vi "LoadPluginRequest.vi"(8 "error in (no error)":errorcluster, 10 "PathToPlugin":path=path "", 11 "ModuleID":i32=-1) -> (0 "error out":errorcluster)   [LabVIEW 2014, in "EventModule.lvlib"]
uses:
  EventModule.lvlib
  clEventType.ctl
  <vilib>/Utility/error.llb/Error Cluster From Error Code.vi
  <vilib>/ErrorRing/Error Ring.xnode
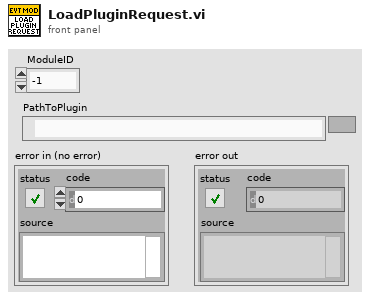
[diagram p1: front panel]
types:
  T1 = typedef "EventModule.lvlib/clRequestEvents.ctl" = cluster{"StopRequest":refnum<user-event>, "LoadPluginRequest":refnum<user-event>, "WriteEvtConfig":refnum<user-event>, "ReadEvtConfig":refnum<user-event>, "WriteTimeArray":refnum<user-event>, "ReadTimeArray":refnum<user-event>, "WriteEvtParams":refnum<user-event>, "ReadEvtParams":refnum<user-event>, "GetEvtReportArray":refnum<user-event>, "ReadPathToPlugin":refnum<user-event>, "GetEvtSignal":refnum<user-event>, "WriteBusNumber":refnum<user-event>, "ReadBusNumber":refnum<user-event>, "ShowPanel":refnum<user-event>}
  T2 = typedef "EventModule.lvlib/clEventType.ctl" = cluster{"ModuleID":i32, "Data":variant}
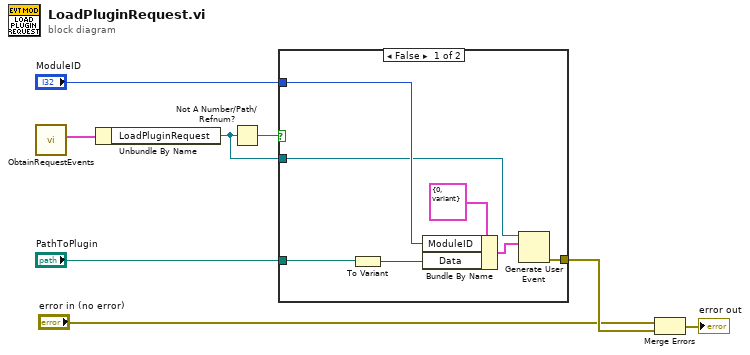
[diagram p0: block diagram]
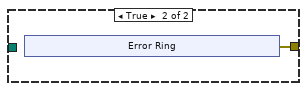
[diagram p2: hidden frame]
diagram:
  n1 = call "ObtainRequestEvents.vi"() -> ("clRequestEvents"=w8:T1)  [unwired: 10 in, 1 out]
  n2 = Unbundle By Name(w8) -> ("LoadPluginRequest"=w6:refnum<user-event>)
  n3 = Not A Number/Path/Refnum?(number/path/refnum=w6) -> (NaN/Path/Refnum?=w7:bool)
  n4 = case shown="False" w7 {
    tunnel: w6 -> [w13 _]
    tunnel: "PathToPlugin" -> [w10 _]
    tunnel: "ModuleID" -> [w14 _]
    tunnel: [w11 w16] -> w2
    frame False {
      n5 = To Variant(anything=w10) -> (Variant=w9:variant)
      n6 = Bundle By Name(cluster=T2 {"ModuleID"=0, "Data"=variant} ("clEventType"), "ModuleID"=w14, "Data"=w9) -> (w12:T2)
      n7 = Generate User Event(user event=w13, event data cluster=w12) -> (error out=w11:errorcluster)  [unwired: 2 in, 1 out]
    }
    frame True {
      n8 = xnode "Error Ring"() -> ("error out"=w16:errorcluster)
    }
  }
  n9 = Merge Errors("error in (no error)", w2) -> (→"error out":errorcluster)
